vi "Read Score Data From File.vi"(10 "XML File Path":path) -> (2 "Array":cluster{"ValidationCount":u16, "Score":T1}[](array[cluster]) {"Score"."Score Mode Selector" items=["Automatic", "Manual"]})   [LabVIEW 2013]
uses:
  Full Score Entry.ctl
  ScoreEntry.ctl
  ScoreList.ctl
  Team Data.ctl
  <vilib>/xml/Close Reference(Node).vi
  <vilib>/xml/NI_XML.lvlib
  <resource>/objmgr/DOMUserDefRef.rc
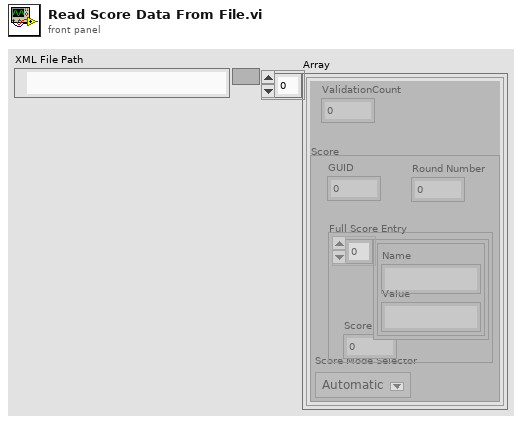
[diagram p1: front panel]
types:
  T1 = typedef "Full Score Entry.ctl" = cluster{"GUID":u16, "Score Mode Selector":u16, "Round Number":u16, "Full Score Entry":T2}
  T2 = typedef "ScoreEntry.ctl" = cluster{"Elements":cluster{"Name":string, "Value":string}[], "Score":dbl}
  T3 = typedef "ScoreList.ctl" = cluster{"ValidationCount":u16, "Score":T1}[]
  T4 = enum16{"Get Teams", "Add Team", "Modify Team", "Clear All Teams", "Force Add Team"}
  T5 = typedef "Team Data.ctl" = cluster{"Both":string, "Name":string, "GUID":u16, "Number":u16}
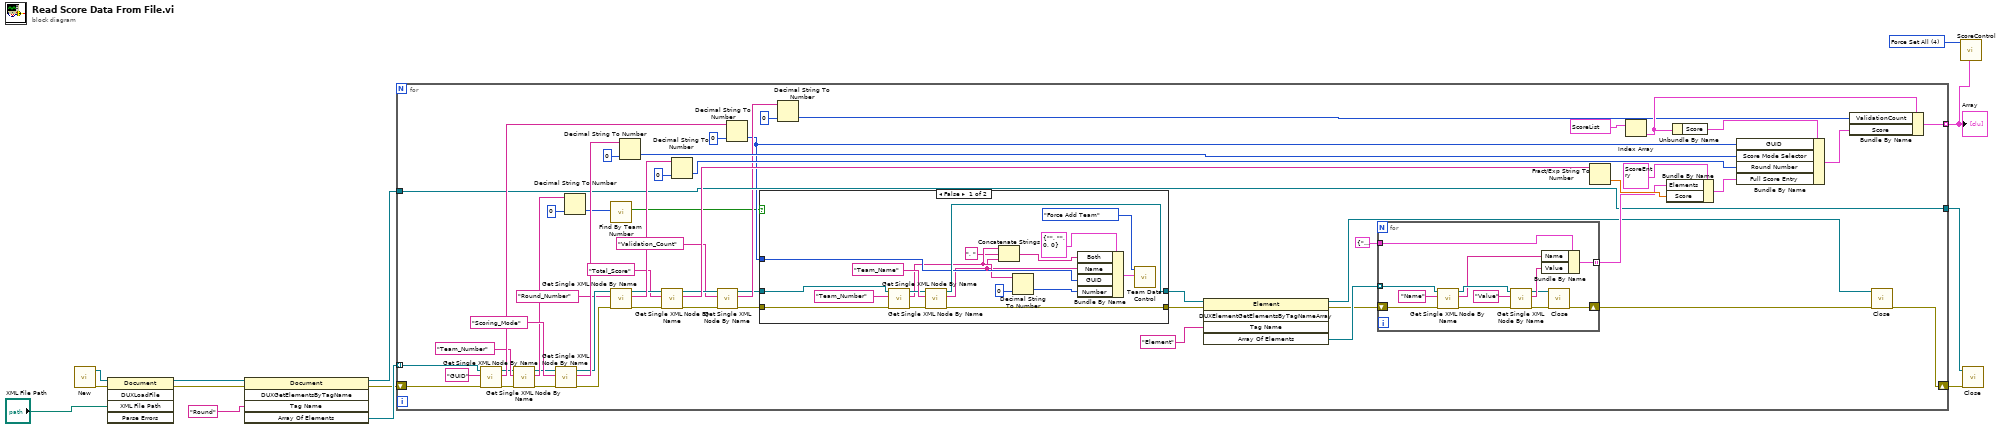
[diagram p0: block diagram]
diagram:
  w2 = u16 4 items=["Get All", "Set", "Reset All", "Force Set", "Force Set All"] ("Get/Set Mode Selector")
  n1 = call <vilib>:"New.vi"() -> ("error out"=w12:errorcluster, "DOM document out"=w13:refnum<k20>)  [unwired: 8 in]
  n2 = invoke class="Document" method="DUXLoadFile"(reference=w13, error in=w12, "XML File Path"="XML File Path") -> (reference out=w10:refnum<k20>, error out=w9:errorcluster)  [unwired: 2 in, 3 out]
  n3 = invoke class="Document" method="DUXGetElementsByTagName"(reference=w10, error in=w9, "Tag Name"="Round") -> (reference out=w4:refnum<k20>, error out=w6:errorcluster, "Array Of Elements"=w7:refnum<k20>[])  [unwired: 2 in, 2 out]
  n4 = for {
    tunnel: w7 -> [w69] mode=indexing
    shift-right: [w41] -> w5
    shift-left: w6 -> [w67]
    tunnel: w4 -> [w39]
    tunnel: [w39] -> w3
    tunnel: [w28] -> w1 mode=indexing
    n5 = call "Get Single XML Node By Name.vi"("error in (no error)"=w67, "Tag Name"="GUID", "Parent Element"=w69) -> ("error out"=w16:errorcluster, "node text"=w66:string, "Parent Element Out"=w17:refnum<k20>)  [unwired: 6 in]
    n6 = call "Get Single XML Node By Name.vi"("error in (no error)"=w16, "Tag Name"="Team_Number", "Parent Element"=w17) -> ("error out"=w14:errorcluster, "node text"=w19:string, "Parent Element Out"=w15:refnum<k20>)  [unwired: 6 in]
    n7 = call "Get Single XML Node By Name.vi"("error in (no error)"=w14, "Tag Name"="Scoring_Mode", "Parent Element"=w15) -> ("error out"=w59:errorcluster, "node text"=w63:string, "Parent Element Out"=w60:refnum<k20>)  [unwired: 6 in]
    n8 = Decimal String To Number(string=w19, default (0L)=u16 0) -> (number=w18:u16)  [unwired: 1 in, 1 out]
    n9 = call "Find By Team Number.vi"("Team Number"=w18) -> ("Found?"=w22:bool)  [unwired: 9 in, 1 out]
    n10 = call "Get Single XML Node By Name.vi"("error in (no error)"=w59, "Tag Name"="Round_Number", "Parent Element"=w60) -> ("error out"=w50:errorcluster, "node text"=w57:string, "Parent Element Out"=w51:refnum<k20>)  [unwired: 6 in]
    n11 = Decimal String To Number(string=w63, default (0L)=u16 0) -> (number=w61:u16)  [unwired: 1 in, 1 out]
    n12 = call "Get Single XML Node By Name.vi"("error in (no error)"=w50, "Tag Name"="Total_Score", "Parent Element"=w51) -> ("error out"=w37:errorcluster, "node text"=w48:string, "Parent Element Out"=w38:refnum<k20>)  [unwired: 6 in]
    n13 = Decimal String To Number(string=w57, default (0L)=u16 0) -> (number=w55:u16)  [unwired: 1 in, 1 out]
    n14 = call "Get Single XML Node By Name.vi"("error in (no error)"=w37, "Tag Name"="Validation_Count", "Parent Element"=w38) -> ("error out"=w25:errorcluster, "node text"=w31:string, "Parent Element Out"=w27:refnum<k20>)  [unwired: 6 in]
    n15 = Decimal String To Number(string=w66, default (0L)=u16 0) -> (number=w23:u16)  [unwired: 1 in, 1 out]
    n16 = case shown="False" w22 {
      tunnel: w27 -> [w81 w89]
      tunnel: [w79 w89] -> w26
      tunnel: w25 -> [w80 w88]
      tunnel: [w78 w88] -> w24
      tunnel: w23 -> [w76 _]
      frame False {
        n17 = call "Get Single XML Node By Name.vi"("error in (no error)"=w80, "Tag Name"="Team_Number", "Parent Element"=w81) -> ("error out"=w84:errorcluster, "node text"=w75:string, "Parent Element Out"=w83:refnum<k20>)  [unwired: 6 in]
        n18 = call "Get Single XML Node By Name.vi"("error in (no error)"=w84, "Tag Name"="Team_Name", "Parent Element"=w83) -> ("error out"=w78:errorcluster, "node text"=w73:string, "Parent Element Out"=w79:refnum<k20>)  [unwired: 6 in]
        n19 = Concatenate Strings(w75, ", ", w73) -> (w72:string)
        n20 = Decimal String To Number(string=w75, default (0L)=u16 0) -> (number=w77:u16)  [unwired: 1 in, 1 out]
        n21 = Bundle By Name(cluster=T5 {"Both"="", "Name"="", "GUID"=0, "Number"=0} ("Team Dataasd"), "Both"=w72, "Name"=w73, "GUID"=w76, "Number"=w77) -> (w71:T5)
        n22 = call "Team Data Control.vi"("Team Data To Add/Change"=w71, "Mode"=T4."Force Add Team") -> ()  [unwired: 9 in, 1 out]
      }
      frame True {
      }
    }
    n23 = Decimal String To Number(string=w31, default (0L)=u16 0) -> (number=w30:u16)  [unwired: 1 in, 1 out]
    n24 = invoke class="Element" method="DUXElementGetElementsByTagNameArray"(reference=w26, error in=w24, "Tag Name"="Element") -> (reference out=w40:refnum<k20>, error out=w45:errorcluster, "Array Of Elements"=w46:refnum<k20>[])  [unwired: 2 in, 2 out]
    n25 = for {
      tunnel: w46 -> [w102] mode=indexing
      shift-right: [w91] -> w42
      shift-left: w45 -> [w101]
      tunnel: cluster{"Name":string, "Value":string} {"Name"="", "Value"=""} -> [w96]
      tunnel: [w90] -> w43 mode=indexing
      n26 = call "Get Single XML Node By Name.vi"("error in (no error)"=w101, "Tag Name"="Name", "Parent Element"=w102) -> ("error out"=w98:errorcluster, "node text"=w95:string, "Parent Element Out"=w99:refnum<k20>)  [unwired: 6 in]
      n27 = call "Get Single XML Node By Name.vi"("error in (no error)"=w98, "Tag Name"="Value", "Parent Element"=w99) -> ("error out"=w92:errorcluster, "node text"=w94:string, "Parent Element Out"=w93:refnum<k20>)  [unwired: 6 in]
      n28 = Bundle By Name(cluster=w96, "Name"=w95, "Value"=w94) -> (w90:cluster{"Name":string, "Value":string})
      n29 = call-poly <vilib>:"Close.vi"("error in (no error)"=w92, "node"=w93) -> ("error out"=w91:errorcluster)  [unwired: 7 in]
    }
    n30 = Fract/Exp String To Number(string=w48) -> (number=w47:dbl)  [unwired: 3 in, 1 out]
    n31 = Index Array(array=T3 [{"ValidationCount"=0, "Score"={"GUID"=0, "Score Mode Selector"=0, "Round Number"=0, "Full Score Entry"={"Elements"=[{"Name"="", "Value"=""}], "Score"=0.0}}}] ("Scores")) -> (element=w33:cluster{"ValidationCount":u16, "Score":T1})  [unwired: 1 in]
    n32 = Bundle By Name(cluster=T2 {"Elements"=[{"Name"="CO2 Balls Touching/Within Reservoir Model", "Value"="-1"}, {"Name"="Money Ball Touching/Within Reservoir Model", "Value"="-1"}, {"Name"="3+ Red/White Citizens in Pink Grid Area", "Value"="-1"}, {"Name"="# Upright Levee Blocks touching ONLY GREEN shores", "Value"="-1"}, {"Name"="# Upright Levee Blocks Touching any RED shore", "Value"="-1"}, {"Name"="Levee Test was Performed", "Value"="-1"}, {"Name"="Levee Test Wheel Blocked by NonLevee", "Value"="-1"}, {"Name"="Flood Barrier in Up Position", "Value"="-1"}, {"Name"="Both Yellow Arrows Aligned", "Value"="-1"}, {"Name"="Team Robot Touching Only Yellow Grid Area", "Value"="-1"}, {"Name"="Both Insulation Touching Green Grid Area", "Value"="-1"}, {"Name"="Bicycle Touching Green Grid Area", "Value"="-1"}, {"Name"="Computer Touching Green Grid Area", "Value"="-1"}, {"Name"="House in Up Position", "Value"="-1"}, {"Name"="House Window Showing Black", "Value"="-1"}, {"Name"="House Window All The Way Open", "Value"="-1"}, {"Name"="3+ Black/White Scientists Touching Research Area", "Value"="-1"}, {"Name"="Money Ball Touching/Within Research Area Model", "Value"="-1"}, {"Name"="Polar Bear Touching/Within Research Area Model", "Value"="-1"}, {"Name"="Polar Bear Orientation (Sleeping/Upright)", "Value"="-1"}, {"Name"="Ice Core Pulled From Its Hole", "Value"="-1"}, {"Name"="Ice Buoy Upright and Within/Touching Research Area Model", "Value"="-1"}, {"Name"="Drilling Machine Touching/Within Research Area Model", "Value"="-1"}, {"Name"="Drill Assembly Completely Vertical", "Value"="-1"}, {"Name"="Team Robot Touching/Within Research Area Model", "Value"="-1"}, {"Name"="3+ Blue/Gray Leaders Touching Green Mountain/City Area", "Value"="-1"}, {"Name"="Ice Core in Base Area", "Value"="-1"}, {"Name"="Snowmobile Touching/Within Research Area Model", "Value"="-1"}], "Score"=0.0} ("Full Score Entry"), "Elements"=w43, "Score"=w47) -> (w52:T2)
    n33 = Unbundle By Name(w33) -> ("Score"=w34:T1)
    n34 = Bundle By Name(cluster=w34, "GUID"=w23, "Score Mode Selector"=w61, "Round Number"=w55, "Full Score Entry"=w52) -> (w32:T1)
    n35 = Bundle By Name(cluster=w33, "ValidationCount"=w30, "Score"=w32) -> (w28:cluster{"ValidationCount":u16, "Score":T1})
    n36 = call-poly <vilib>:"Close.vi"("error in (no error)"=w42, "node"=w40) -> ("error out"=w41:errorcluster)  [unwired: 7 in]
  }
  "Array" <- w1
  n37 = call "ScoreControl.vi"("Get/Set Mode Selector"=w2, "All Scores"=w1) -> ()  [unwired: 12 in, 2 out]
  n38 = call-poly <vilib>:"Close.vi"("error in (no error)"=w5, "node"=w3) -> ()  [unwired: 7 in, 1 out]
